vi "Calculate Terminal Size.vi"(8 "error in (no error)":errorcluster, 11 "Terminal in":refnum<class "Terminal.lvclass">) -> (0 "error out":errorcluster, 2 "Terminal Size":cluster{"Cols":u32, "Rows":u32}, 3 "Terminal out":refnum<class "Terminal.lvclass">)   [LabVIEW 2020, in "Terminal.lvlib" / "Terminal.lvclass"]
uses:
  Terminal.lvclass
  Terminal.lvclass/Terminal.ctl
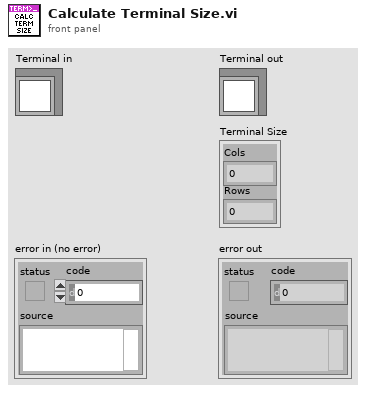
[diagram p1: front panel]
types:
  T1 = typedef "Terminal.lvlib/Terminal.lvclass/Ref Data.ctl" = cluster{"Connection":refnum<class "Connection.lvclass">, "Read Loop Running":bool, "Parse State":T2, "Terminal Options":T7, "Font Metrics":T10}
  T2 = typedef "Terminal.lvlib/Terminal.lvclass/Parse State.ctl" = cluster{"Buffer State":T3, "Cursor":T4, "Attributes":T6}
  T3 = typedef "Terminal.lvlib/Terminal.lvclass/Buffer State.ctl" = cluster{"Sequence":string, "ESC":bool, "Alt Buf":bool}
  T4 = typedef "Terminal.lvlib/Terminal.lvclass/Cursor.ctl" = cluster{"Cur":T5, "Saved":T5}
  T5 = typedef "Terminal.lvlib/Terminal.lvclass/Position.ctl" = cluster{"Row":i32, "Col":i32}
  T6 = typedef "Terminal.lvlib/Text Attributes.ctl" = cluster{"FG":u32, "BG":u32, "Bold":bool, "Italic":bool, "Underline":bool, "Strike":bool, "Inverse":bool}
  T7 = typedef "Terminal.lvlib/Terminal Options.ctl" = cluster{"Implied CR with LF":bool, "Local Echo":bool, "Tab Width":i32, "Color Scheme":T8, "Default FG":T9, "Default BG":T9, "History Length":i32, "Font Face":string, "Font Size":i16, "Rows":i32, "Cols":i32}
  T8 = typedef "Terminal.lvlib/Color Scheme.ctl" = cluster{"Black":u32, "Red":u32, "Green":u32, "Yellow":u32, "Blue":u32, "Magenta":u32, "Cyan":u32, "White":u32, "Bright Black":u32, "Bright Red":u32, "Bright Green":u32, "Bright Yellow":u32, "Bright Blue":u32, "Bright Magenta":u32, "Bright Cyan":u32, "Bright White":u32}
  T9 = typedef "Terminal.lvlib/Color.ctl" = i8
  T10 = typedef "Terminal.lvlib/Terminal.lvclass/Font Metrics.ctl" = cluster{"Width":i16, "Height":i16}
  T11 = typedef "LVBoundsTypeDef.ctl" = cluster{"Width":u32, "Height":u32}
  T12 = enum16{"User-specified Font", "Application Font", "System Font", "Dialog Font"}
  T13 = cluster{"Font Name:":string, "Size":i16, "Strikeout?":bool, "Italic?":bool, "Underline?":bool, "Outline?":bool, "Shadow?":bool, "Bold?":bool}
  T14 = cluster{"left":i16, "top":i16, "right":i16, "bottom":i16}
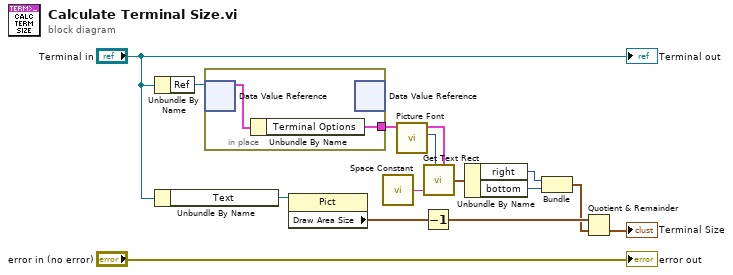
[diagram p0: block diagram]
diagram:
  n1 = Unbundle By Name("Terminal in") -> ("Ref"=w13:refnum<data-value>)
  n2 = Unbundle By Name("Terminal in") -> ("Text"=w14:refnum<vi>)
  n3 = in-place {
    in-place-border: [w16] -> w12
    n4 = in-place-dvr #1(w13) -> (w17:T1)  [unwired: 1 out]
    n5 = Unbundle By Name(w17) -> ("Terminal Options"=w16:T7)
    n6 = in-place-dvr #1() -> ()  [unwired: 1 in, 2 out]
  }
  n7 = property class="Pict"(reference=w14) -> ("Draw Area Size"=w8:T11)  [unwired: 1 in, 2 out]
  n8 = call <vilib>:"Space Constant.vi"() -> ("String"=w9:string)
  n9 = call "Picture Font.vi"("Terminal Options"=w12) -> ("desired font"=w10:T12, "Picture Font"=w11:T13)  [unwired: 7 in, 2 out]
  n10 = Decrement(x=w8) -> (x-1=w7:T11)
  n11 = call <vilib>:"Get Text Rect.vi"("desired font(Application)"=w10, "text"=w9, "[user-specified font]"=w11) -> ("rect"=w6:T14)  [unwired: 6 in]
  n12 = Unbundle By Name(w6) -> ("right"=w4:i16, "bottom"=w5:i16)
  n13 = Bundle("right"=w4, "bottom"=w5) -> (w3:cluster{"right":i16, "bottom":i16})  [unwired: 1 in]
  n14 = Quotient & Remainder(x=w7, y=w3) -> (floor(x/y)=→"Terminal Size":T11)  [unwired: 1 out]
  "error out" <- "error in (no error)"
  "Terminal out" <- "Terminal in"
